vi "add method by path.vi"(6 "parameters":variant[](array[variant]), 8 "error in":errorcluster, 9 "exclusions":string[](array[string]), 10 "Path":path, 11 "vi modification tool in":refnum<class "vi modification tool.lvclass">) -> (0 "error out":errorcluster, 3 "vi modification tool out":refnum<class "vi modification tool.lvclass">)   [LabVIEW 2013, in "vi modification tool.lvclass"]
uses:
  vi modification tool.lvclass
  method call.ctl
  vi modification tool.lvclass/vi modification tool.ctl
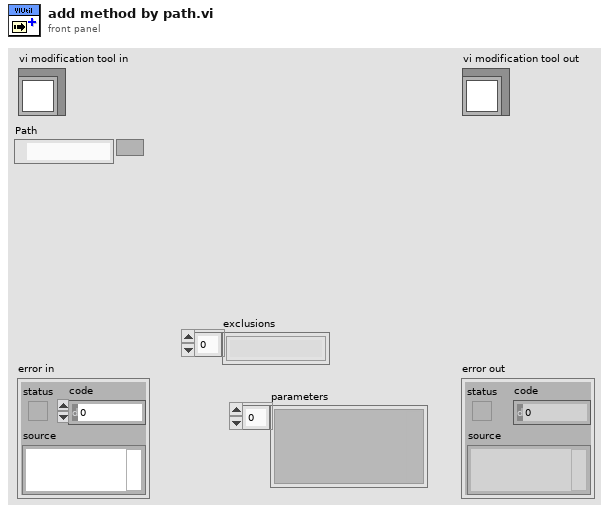
[diagram p1: front panel]
types:
  T1 = typedef "vi modification tool.lvclass/method call.ctl" = cluster{"Path":path, "parameters":variant[], "exclusions":string[]}
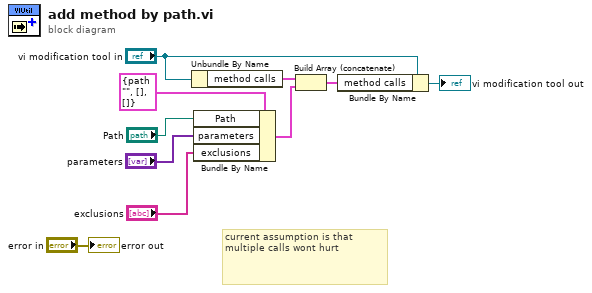
[diagram p0: block diagram]
diagram:
  # "current assumption is that multiple calls wont hurt"
  n1 = Unbundle By Name("vi modification tool in") -> ("method calls"=w3:T1[])
  n2 = Bundle By Name(cluster=T1 {"Path"=path "", "parameters"=[], "exclusions"=[]} ("method call"), "Path"="Path", "parameters"="parameters", "exclusions"="exclusions") -> (w6:T1)
  n3 = Build Array (concatenate)(w3, w6) -> (w2:T1[])
  n4 = Bundle By Name(cluster="vi modification tool in", "method calls"=w2) -> (→"vi modification tool out":refnum<class "vi modification tool.lvclass">)
  "error out" <- "error in"
